vi "Dataflow.vi"() -> ()   [LabVIEW 2010]
doc: "A sample VI used to demonstrate dataflow."
panel:
  out "C 2":dbl
  in  "A 2":dbl
  out "C":dbl
  in  "B":dbl min=0.0 max=100.0 step=1.0
  in  "A":dbl
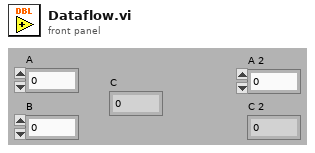
[diagram p1: front panel]
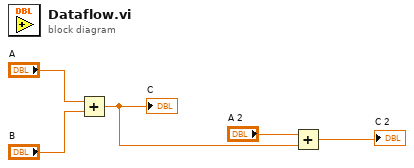
[diagram p0: block diagram]
diagram:
  n1 = Add(x="A", y="B") -> (x+y=w2:dbl)
  "C" <- w2
  n2 = Add(x="A 2", y=w2) -> (x+y=→"C 2":dbl)
